vi "Read Transport.vi"(11 "ISubscriptionPolicy in":refnum<class "ISubscriptionPolicy.lvclass">) -> (2 "Transport":refnum<class "ITransport.lvclass">)   [LabVIEW 2015, in "IMediator.lvlib" / "ISubscriptionPolicy.lvclass"]
uses:
  ISubscriptionPolicy.lvclass
  ITransport/ITransport.lvclass
  ISubscriptionPolicy.lvclass/ISubscriptionPolicy.ctl
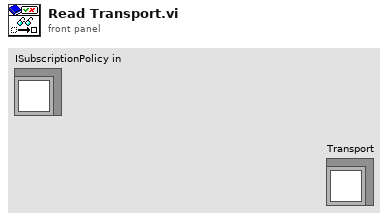
[diagram p1: front panel]
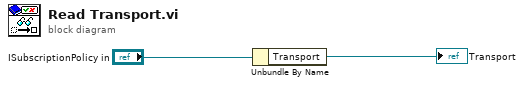
[diagram p0: block diagram]
diagram:
  n1 = Unbundle By Name("ISubscriptionPolicy in") -> ("Transport"=→"Transport":refnum<class "ITransport.lvclass">)
